vi "COM Disconnect.vi"(6 "VISA resource name":refnum<visa-resource-name>, 8 "Error In":errorcluster, 11 "Connection Status":T1) -> (0 "Error Out":errorcluster, 3 "Connection Status":T1, 4 "VISA resource name":refnum<visa-resource-name>)   [LabVIEW 2014]
doc: "Disconnects COM Port"
uses:
  Controls/Connection Status.ctl
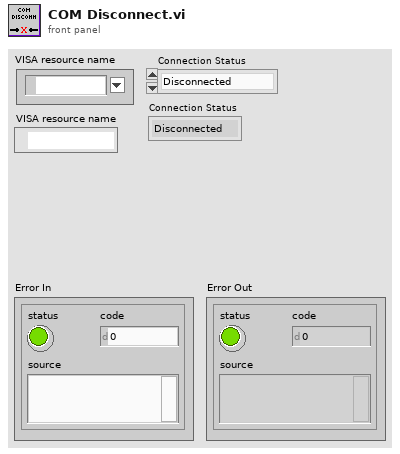
[diagram p1: front panel]
types:
  T1 = typedef "Connection Status.ctl" = enum16{"Disconnected", "Connected"}
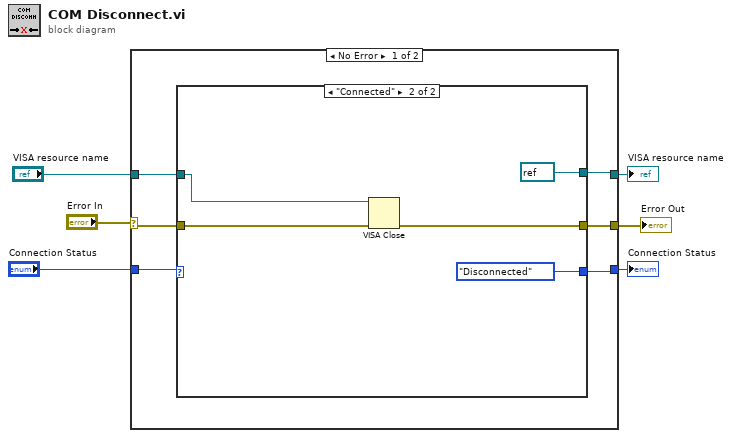
[diagram p0: block diagram]
diagram:
  n1 = case shown="No Error" "Error In" {
    selector: "Error In" -> [w11 w23]
    tunnel: "VISA resource name" -> [w9 w22]
    tunnel: "Connection Status" -> [w12 w21]
    tunnel: [w10 w23] -> w3
    tunnel: [w8 w22] -> w2
    tunnel: [w7 w21] -> w1
    frame No Error {
      n2 = case shown="\"Connected\"" w12 {
        selector: w12 -> [w14 _]
        tunnel: w11 -> [w15 w20]
        tunnel: [w15 w19] -> w10
        tunnel: w9 -> [w13 w18]
        tunnel: [w13 refnum<visa-resource-name> refnum ("VISA resource name")] -> w8
        tunnel: [w14 Connection_Status."Disconnected" ("Connection Status")] -> w7
        frame "Disconnected" {
          # "If Disconnected do nothing"
        }
        frame "Connected" {
          n3 = VISA Close(VISA resource name=w18, error in (no error)=w20) -> (error out=w19:errorcluster)
        }
      }
    }
    frame Error {
    }
  }
  "Error Out" <- w3
  "VISA resource name" <- w2
  "Connection Status" <- w1
